vi "Module-error.vi"(8 "error in (no error)":errorcluster, 10 "Error":T1) -> (0 "error out":errorcluster)   [LabVIEW 2013, in "SettingsFile.lvlib" / "SettingsFile.lvclass"]
uses:
  SettingsFile.lvclass
  Errors.ctl
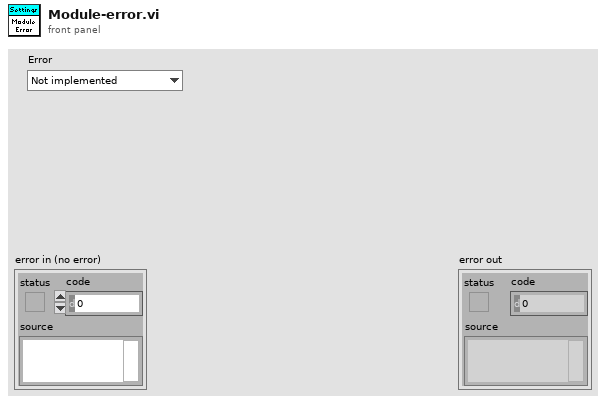
[diagram p1: front panel]
types:
  T1 = typedef "SettingsFile.lvlib/SettingsFile.lvclass/Errors.ctl" = enum16{"Not implemented", "Command not recognized", "Invalid input", "No connection", "Timeout", "Invalid file type", "No file access"}
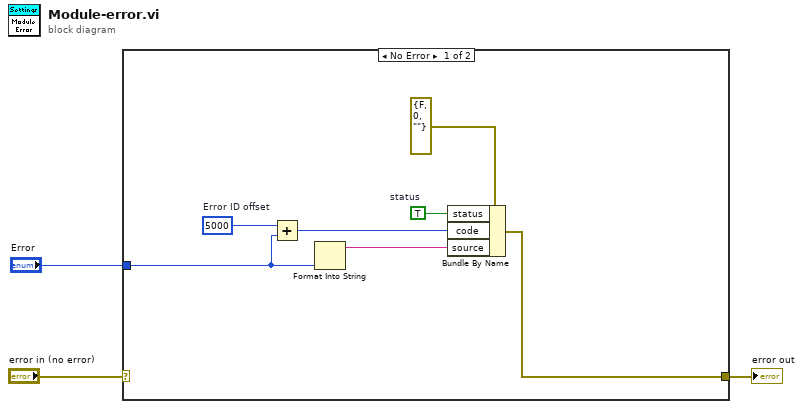
[diagram p0: block diagram]
diagram:
  n1 = case shown="No Error" "error in (no error)" {
    selector: "error in (no error)" -> [_ w11]
    tunnel: [w4 w11] -> w2
    tunnel: "Error" -> [w10 _]
    frame No Error {
      w5 = TRUE  # status
      w9 = 5000  # Error ID offset
      n2 = Add(x=w9, y=w10) -> (x+y=w6:i32)
      n3 = Format Into String(w10) -> (resulting string=w7:string)  [unwired: 3 in, 1 out]
      n4 = Bundle By Name(cluster=errorcluster {"status"=FALSE, "code"=0, "source"=""} ("error constant"), "status"=w5, "code"=w6, "source"=w7) -> (w4:errorcluster)
    }
    frame Error {
    }
  }
  "error out" <- w2
